vi "draw png at point.vi"(8 "top left point(0, 0)":cluster{"x":i16, "y":i16}, 10 "image data":T1, 11 "new picture in":picture) -> (3 "new picture out":picture)   [LabVIEW 2023]
uses:
  <vilib>/picture/picture.llb/imagedata.ctl
  <vilib>/picture/picture.llb/Draw True-Color Pixmap.vi
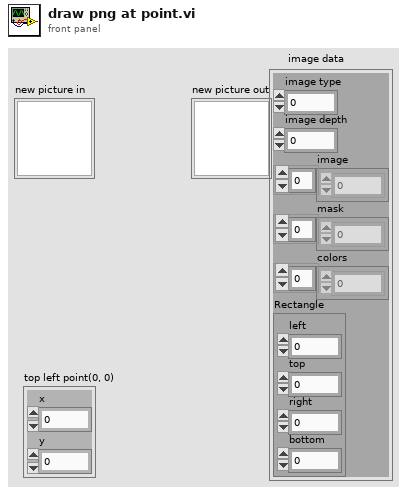
[diagram p1: front panel]
types:
  T1 = typedef "imagedata.ctl" = cluster{"image type":i32, "image depth":i32, "image":u8[], "mask":u8[], "colors":u32[], "Rectangle":cluster{"left":i16, "top":i16, "right":i16, "bottom":i16}}
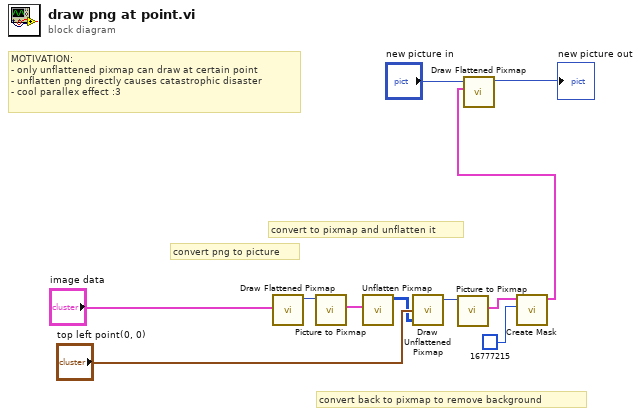
[diagram p0: block diagram]
diagram:
  # "convert back to pixmap to remove background"
  # "MOTIVATION:\n- only unflattened pixmap can draw at certain point\n- unflatten png directly causes catastrophic disaster\n- cool parallex effect :3"
  # "convert to pixmap and unflatten it"
  # "convert png to picture"
  n1 = call <vilib>:"Draw Flattened Pixmap.vi"("image data"="image data") -> ("new picture"=w2:picture)  [unwired: 8 in]
  n2 = call <vilib>:"Picture to Pixmap.vi"("picture"=w2) -> ("image data"=w6:T1)  [unwired: 9 in, 1 out]
  n3 = call <vilib>:"Unflatten Pixmap.vi"("image data"=w6) -> ("24-bit pixmap"=w3:u32[][])  [unwired: 4 in, 6 out]
  n4 = call-poly <vilib>:"Draw Unflattened Pixmap.vi"("top left point(0, 0)"="top left point(0, 0)", "data (RGB format)"=w3) -> ("new picture"=w5:picture)  [unwired: 7 in]
  n5 = call <vilib>:"Picture to Pixmap.vi"("picture"=w5) -> ("image data"=w7:T1)  [unwired: 9 in, 1 out]
  n6 = call <vilib>:"Create Mask.vi"("Mask Color (Black)"=u32 16777215, "image data"=w7) -> ("image data"=w10:T1)  [unwired: 9 in]
  n7 = call <vilib>:"Draw Flattened Pixmap.vi"("image data"=w10, "picture"="new picture in") -> ("new picture"=→"new picture out":picture)  [unwired: 7 in]
